vi "Score_For_Door.vi"(8 "error in (no error)":errorcluster, 11 "Door":T1) -> (0 "error out":errorcluster, 3 "Score":i32)   [LabVIEW 2026]
uses:
  Controls/Door_Status_Enum.ctl
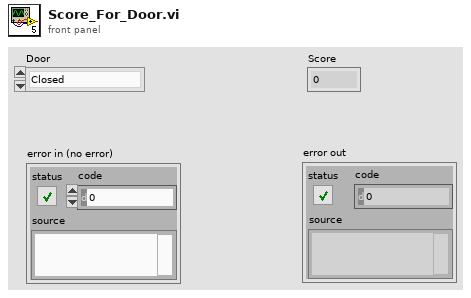
[diagram p1: front panel]
types:
  T1 = typedef "Door_Status_Enum.ctl" = enum16{"Closed", "Open", "Opening", "Closing"}
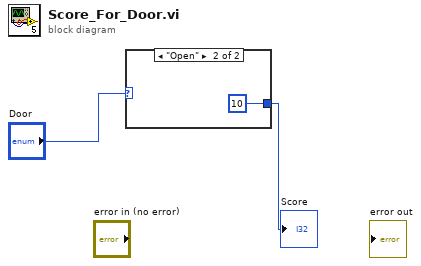
[diagram p0: block diagram]
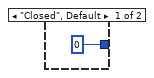
[diagram p2: hidden frame]
diagram:
  n1 = case shown="\"Open\"" "Door" {
    tunnel: [0 10] -> w2
    frame "Closed", Default {
    }
    frame "Open" {
    }
  }
  "Score" <- w2
